vi "FMA1600A Initialize.vi"(7 "baud rate (9600)":u32=19200, 8 "error in (no error)":errorcluster, 11 "VISA Refnum in":refnum<visa-resource-name>) -> (0 "error out":errorcluster, 3 "VISA Refnum out":refnum<visa-resource-name>)   [LabVIEW 2016]
uses:
  <vilib>/Instr/_visa.llb/VISA Open Access Mode.ctl
  <vilib>/Instr/_visa.llb/VISA Configure Serial Port (Instr).vi
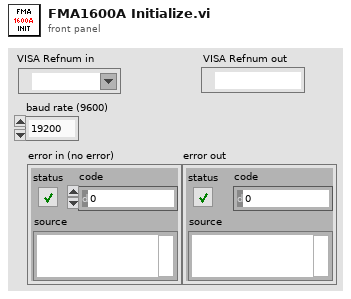
[diagram p1: front panel]
types:
  T1 = typedef "VISA Open Access Mode.ctl" = u32
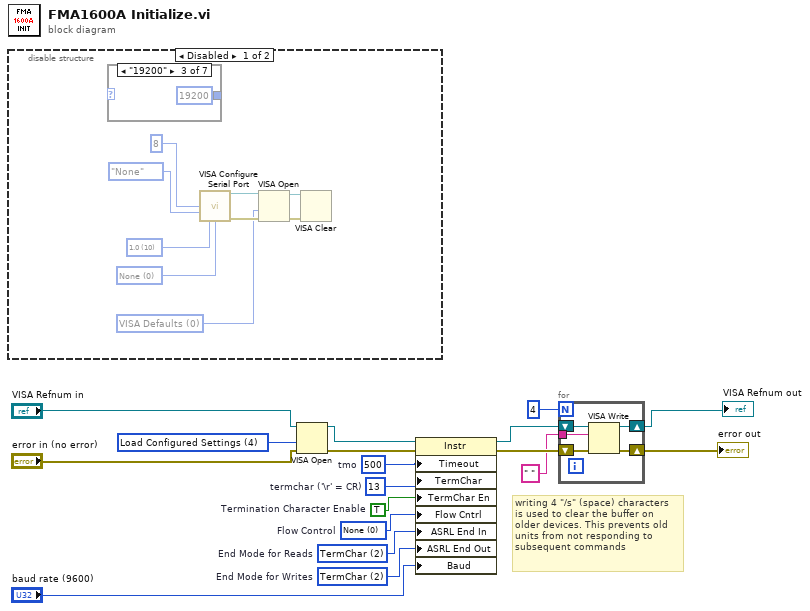
[diagram p0: block diagram]
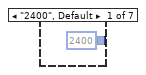
[diagram p2: hidden frame]
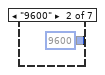
[diagram p3: hidden frame]
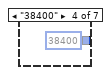
[diagram p4: hidden frame]
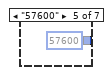
[diagram p5: hidden frame]
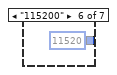
[diagram p6: hidden frame]
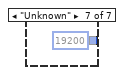
[diagram p7: hidden frame]
diagram:
  w8 = T1 4 items=["VISA Defaults"=0, "Exclusive Lock"=1, "Load Configured Settings"=4] ("Access Mode")
  w9 = u32 500  # tmo
  w10 = u16 2 items=["None", "Last Bit", "TermChar", "Break"]  # End Mode for Writes
  w11 = u16 2 items=["None", "Last Bit", "TermChar"]  # End Mode for Reads
  w12 = u16 0 items=["None", "XON/XOFF", "RTS/CTS", "XON/XOFF & RTS/CTS", "DTR/DSR", "XON/XOFF & DTR/DSR"]  # Flow Control
  w13 = TRUE  # Termination Character Enable
  w14 = u8 13  # termchar ('\r' = CR)
  # "writing 4 \"/s\" (space) characters\nis used to clear the buffer on \nolder devices. This prevents old\nunits from not responding to \nsubsequent commands"
  n1 = disable-structure shown="Disabled" {
    frame Disabled {
      w19 = T1 0 items=["VISA Defaults"=0, "Exclusive Lock"=1, "Load Configured Settings"=4] ("Access Mode")
      w24 = u16 0 items=["None", "XON/XOFF", "RTS/CTS", "XON/XOFF & RTS/CTS", "DTR/DSR", "XON/XOFF & DTR/DSR"] ("flow control (0:none)")
      w25 = u16 10 items=["1.0"=10, "1.5"=15, "2.0"=20] ("stop bits (10: 1 bit)")
      n2 = case shown="\"19200\"" {
        selector: _ -> [_ _ _ _ _ _ _]
        tunnel: [u32 2400 ("Serial Settings:Baud Rate") u32 9600 ("Serial Settings:Baud Rate") u32 19200 ("Serial Settings:Baud Rate") u32 38400 ("Serial Settings:Baud Rate") u32 57600 ("Serial Settings:Baud Rate") u32 11520 ("Serial Settings:Baud Rate") u32 19200 ("Serial Settings:Baud Rate")] -> _
        frame "2400", Default {
        }
        frame "9600" {
        }
        frame "19200" {
        }
        frame "38400" {
        }
        frame "57600" {
        }
        frame "115200" {
        }
        frame "Unknown" {
        }
      }
      n3 = call-poly "VISA Configure Serial Port"("data bits (8)"=u16 8, "parity (0:none)"=enum16{"None", "Odd", "Even", "Mark", "Space"}."None", "stop bits (10: 1 bit)"=w25, "flow control (0:none)"=w24) -> ("VISA resource name out"=w21:refnum<visa-resource-name>, "error out"=w20:errorcluster)  [unwired: 10 in]
      n4 = VISA Open(access mode=w19, error in (no error)=w20, VISA resource name=w21) -> (VISA resource name=w22:refnum<visa-resource-name>, error out=w23:errorcluster)  [unwired: 2 in]
      n5 = VISA Clear(VISA resource name=w22, error in (no error)=w23) -> ()  [unwired: 2 out]
    }
    frame Enabled {
    }
  }
  n6 = VISA Open(access mode=w8, error in (no error)="error in (no error)", VISA resource name="VISA Refnum in") -> (VISA resource name=w7:refnum<visa-resource-name>, error out=w6:errorcluster)  [unwired: 2 in]
  n7 = property class="Instr"(reference=w7, error in=w6, "Timeout"=w9, "TermChar"=w14, "TermChar En"=w13, "Flow Cntrl"=w12, "ASRL End In"=w11, "ASRL End Out"=w10, "Baud"="baud rate (9600)") -> (reference out=w18:refnum<visa-resource-name>, error out=w17:errorcluster)
  n8 = for {
    N: 4 -> [_]
    tunnel: " " -> [w35]
    shift-right: [w36] -> w4
    shift-left: w18 -> [w37]
    shift-right: [w38] -> w3
    shift-left: w17 -> [w39]
    n9 = VISA Write(VISA resource name=w37, write buffer=w35, error in (no error)=w39) -> (VISA resource name out=w36:refnum<visa-resource-name>, error out=w38:errorcluster)  [unwired: 1 out]
  }
  "VISA Refnum out" <- w4
  "error out" <- w3
